vi "setEndpointElement.vi"(8 "error in (no error)":errorcluster, 9 "Value":string, 10 "Endpoint Name":string, 11 "Oauth2 in":refnum<class "Oauth2.lvclass">) -> (0 "error out":errorcluster, 3 "Oauth2 out":refnum<class "Oauth2.lvclass">)   [LabVIEW 2020, in "Oauth2.lvclass"]
uses:
  Oauth2.lvclass
  Oauth2.lvclass/Oauth2.ctl
  OAuthToken/OAuthAccessToken.lvclass
  OAuthToken/OAuth2 Token Element -- enum.ctl
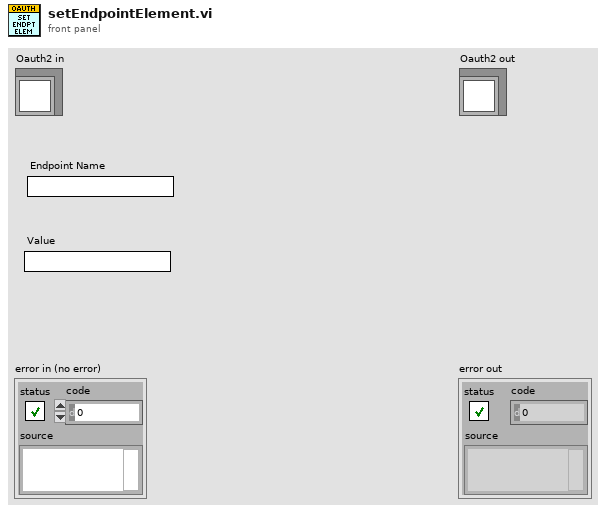
[diagram p1: front panel]
types:
  T1 = typedef "OAuthAccessToken.lvclass/OAuth2 Token Element -- enum.ctl" = enum16{"client_id", "client_secret", "response_type", "scope", "redirect_uri", "error", "error_description", "error_uri", "grant_type", "code", "access_token", "token_type", "expires_in", "username", "password", "refresh_token", "code_challenge", "code_challenge_method", "reverse_proxy_uri", "endpoint element"}
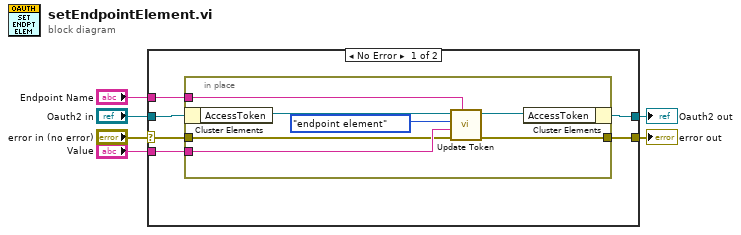
[diagram p0: block diagram]
diagram:
  n1 = case shown="No Error" "error in (no error)" {
    selector: "error in (no error)" -> [w9 w21]
    tunnel: [w8 w21] -> w5
    tunnel: [w11 w20] -> w3
    tunnel: "Oauth2 in" -> [w12 w20]
    tunnel: "Value" -> [w10 _]
    tunnel: "Endpoint Name" -> [w7 _]
    frame No Error {
      n2 = in-place {
        in-place-border: w10 -> [w16]
        in-place-border: w9 -> [w15]
        in-place-border: [w14] -> w8
        in-place-border: w7 -> [w13]
        n3 = in-place-cluster #1(w12) -> ("AccessToken"=w19:refnum<class "OAuthAccessToken.lvclass">)
        n4 = call "Update Token.vi"("Endpoint element key"=w13, "error in (no error)"=w15, "Value"=w16, "Token element"=OAuth2_Token_Element_--_enum."endpoint element", "OAuthAccessToken in"=w19) -> ("error out"=w14:errorcluster, "OAuthAccessToken out"=w18:refnum<class "OAuthAccessToken.lvclass">)  [unwired: 5 in]
        n5 = in-place-cluster #1("AccessToken"=w18) -> (w11:refnum<class "Oauth2.lvclass">)
      }
    }
    frame Error {
    }
  }
  "error out" <- w5
  "Oauth2 out" <- w3
